vi "Init.vi"(6 "Registration":refnum<event-registration>, 8 "Queue Mailbox":refnum<data-value>, 9 "Self Event":refnum<data-value>, 10 "Self Event Alias":string) -> (3 "Base Event out":refnum<class "Base Event.lvclass">)   [LabVIEW 2021, in "jettl.lvlib" / "Base Event.lvlib" / "Base Event.lvclass"]
uses:
  Base Event.lvclass
  Base Event.lvclass/Base Event.ctl
  State/Nominal State/Nominal State.lvclass
  C:/git/jettl/jettl/jettl/Base Event/State/State/State.lvclass
  Addresses/Addresses/Addresses.lvclass
  Msg Strategy/Msg Strategy.lvclass
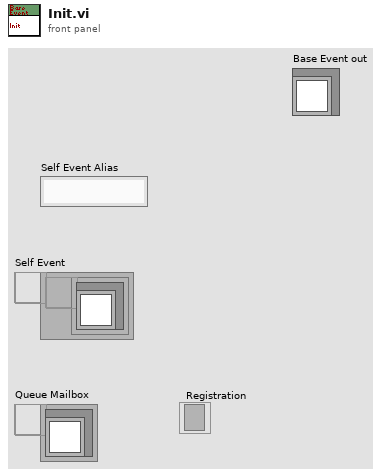
[diagram p1: front panel]
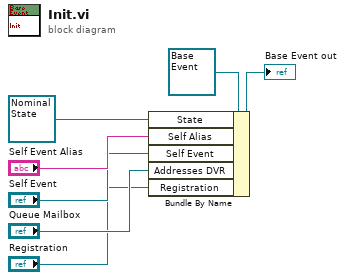
[diagram p0: block diagram]
diagram:
  n1 = Bundle By Name(cluster=refnum<class "Base Event.lvclass"> refnum ("jettl Event Actor out"), "State"=refnum<class "Nominal State.lvclass"> refnum ("jettl.lvlib:Nominal Event State.lvclass"), "Self Alias"="Self Event Alias", "Self Event"="Self Event", "Addresses DVR"="Queue Mailbox", "Registration"="Registration") -> (→"Base Event out":refnum<class "Base Event.lvclass">)
